vi "Configure Measurement Characteristics.vi"(0 "VISA resource name":refnum<visa-resource-name>, 1 "Input Measurement Type (2: Average Power)":i32(ring)=2 items=["Peak Power", "Peak to Average Power", "Average Power", "Minimum Power"], 2 "Measurement Type (0: Sensor1)":i32(ring) items=["Sensor1", "Sensor1-Sensor1", "Sensor1/Sensor1"], 5 "Measurement Rate (0: Normal)":i32(ring) items=["Normal", "Double", "Fast"], 7 "Calculate Block (1: Calculate Block 1)":i32(ring)=1 items=["Calculate Block 1"=1, "Calculate Block 2"=2, "Calculate Block 3"=3, "Calculate Block 4"=4], 9 "Resolution (1)":dbl=1.0, 11 "error in (no error)":errorcluster, 12 "Sweep (0: No Sweep)":i32(ring) items=["No Sweep", "Sweep1", "Sweep2", "Sweep3", "Sweep4"], 13 "Expected Value (0)":dbl) -> (4 "VISA resource name out":refnum<visa-resource-name>, 15 "error out":errorcluster)   [LabVIEW 2014, in "Agilent U2000 Series.lvlib"]
doc: "Configures the instrument to take single or dual channel measurements. \n\nNote:\nThis VI supports model U2020 X-Series and U2040 X-Series only."
uses:
  Agilent U2000 Series.lvlib
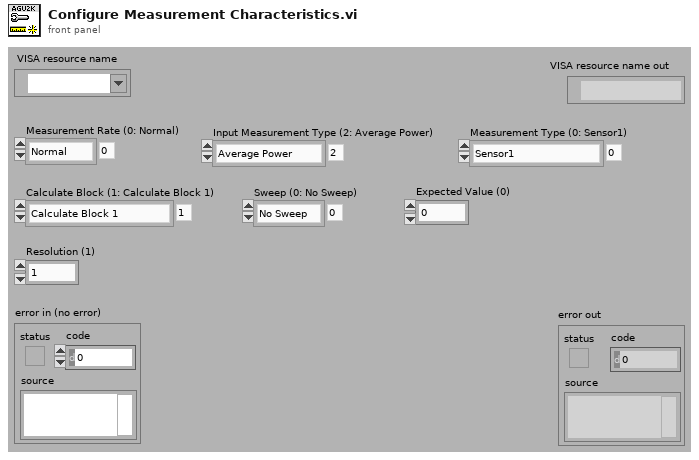
[diagram p1: front panel]
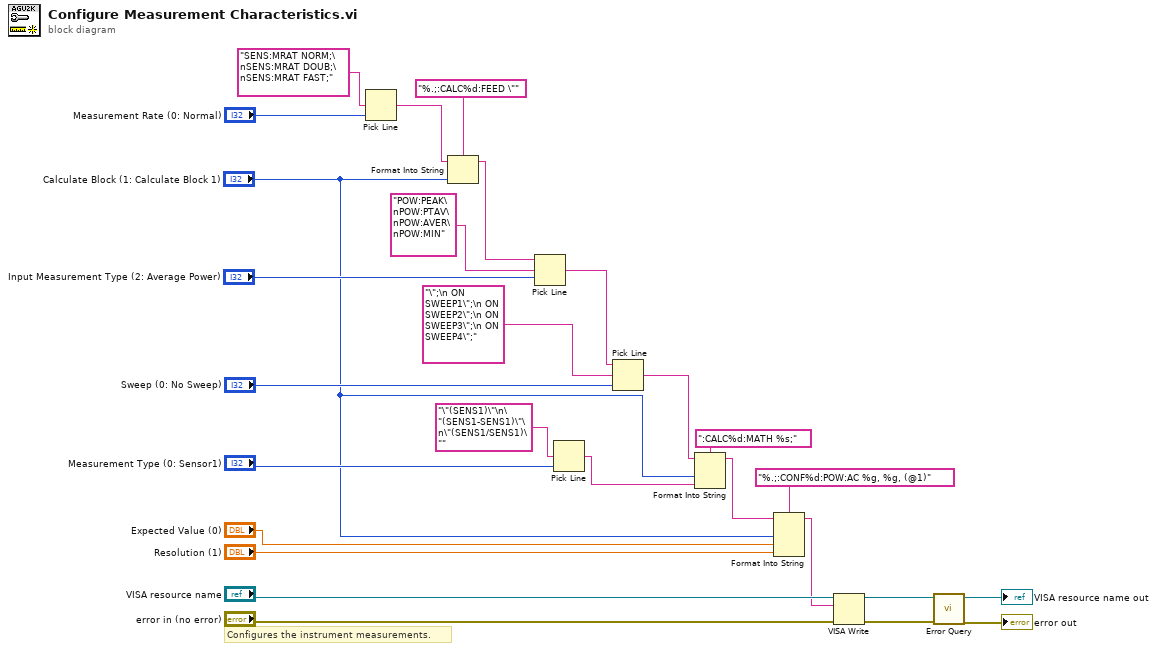
[diagram p0: block diagram]
diagram:
  # "Configures the instrument measurements."
  n1 = Pick Line(multi-line string="SENS:MRAT NORM;\nSENS:MRAT DOUB;\nSENS:MRAT FAST;", line index="Measurement Rate (0: Normal)") -> (output string=w14:string)  [unwired: 1 out]
  n2 = Format Into String(format string="%.;:CALC%d:FEED \"", initial string=w14, "Calculate Block (1: Calculate Block 1)") -> (resulting string=w12:string)  [unwired: 1 in, 1 out]
  n3 = Pick Line(string ("")=w12, multi-line string="POW:PEAK\nPOW:PTAV\nPOW:AVER\nPOW:MIN", line index="Input Measurement Type (2: Average Power)") -> (output string=w9:string)
  n4 = Pick Line(multi-line string="\"(SENS1)\"\n\"(SENS1-SENS1)\"\n\"(SENS1/SENS1)\"", line index="Measurement Type (0: Sensor1)") -> (output string=w21:string)  [unwired: 1 out]
  n5 = Pick Line(string ("")=w9, multi-line string="\";\n ON SWEEP1\";\n ON SWEEP2\";\n ON SWEEP3\";\n ON SWEEP4\";", line index="Sweep (0: No Sweep)") -> (output string=w7:string)
  n6 = Format Into String(format string=":CALC%d:MATH %s;", initial string=w7, "Calculate Block (1: Calculate Block 1)", w21) -> (resulting string=w6:string)  [unwired: 1 in, 1 out]
  n7 = Format Into String(format string="%.;:CONF%d:POW:AC %g, %g, (@1)", initial string=w6, "Calculate Block (1: Calculate Block 1)", "Expected Value (0)", "Resolution (1)") -> (resulting string=w1:string)  [unwired: 1 in, 1 out]
  n8 = VISA Write(VISA resource name="VISA resource name", write buffer=w1, error in (no error)="error in (no error)") -> (VISA resource name out=w18:refnum<visa-resource-name>, error out=w17:errorcluster)  [unwired: 1 out]
  n9 = call "Error Query.vi"("error in (no error)"=w17, "VISA resource name"=w18) -> ("error out"=→"error out":errorcluster, "VISA resource name out"=→"VISA resource name out":refnum<visa-resource-name>)  [unwired: 8 out]
